vi "BALL-AND-BEAM.vi"() -> ()   [LabVIEW 2021]
uses:
  <vilib>/addons/control/pid/pid.llb/PID Structure.ctl
  <vilib>/addons/control/pid/pid.llb/PID Gain Unit.ctl
  <vilib>/addons/control/pid/pid.llb/PID Time Unit.ctl
  <vilib>/MakerHub/LINX/Public/Utilities/Open Serial.vi
  <vilib>/MakerHub/LINX/Public/Sensors/Motion/Servo/Servo Open One Channel.vi
  <vilib>/addons/control/pid/pid.llb/PID Structure Conversion (DBL).vi
  <vilib>/addons/control/pid/pid.llb/PID Advanced (DBL).vi
  <vilib>/MakerHub/LINX/Public/Sensors/Motion/Servo/Servo Set Pulse Width One Channel.vi
  <vilib>/MakerHub/LINX/Public/Sensors/Motion/Servo/Servo Close One Channel.vi
  <vilib>/MakerHub/LINX/LMH-LINX.lvlib
  <vilib>/MakerHub/LINX/Public/Sensors/Motion/Servo/Servo.lvlib
  <vilib>/MakerHub/LINX/Public/Sensors/Distance/Ultrasonic/Ultrasonic.lvlib
  <vilib>/ptbypt/NI_PtbyPt.lvlib
  <vilib>/addons/control/pid/NI_PID_pid.lvlib
panel:
  in  "auto? (T)":bool=TRUE
  out "XY Graph":cluster{"X":dbl, "Y":dbl}[](graph)
  in  "reinitialize? (F)":bool
  in  "manual control":dbl format="%.2f"
  out "BALL STABLE?":bool
  in  "output range":cluster{"output high":dbl, "output low":dbl}={"output high"=100.0, "output low"=-100.0} {"output low" format="%.2f"; "output high" format="%.2f"}
  out "Waveform Chart":cluster{"Dist":dbl, "Set Point":dbl}(graph)
  in  "setpoint range":cluster{"setpoint high":dbl, "setpoint low":dbl}={"setpoint high"=100.0, "setpoint low"=0.0} {"setpoint high" format="%.2f"; "setpoint low" format="%.2f"}
  out "PID OUTPUT":dbl
  in  "derivative unit":T1 items=["min", "s"]
  in  "integral unit":T1 items=["min", "s"]
  in  "derivative":dbl
  in  "integral":dbl
  in  "proportional":dbl
  in  "proportional unit":T2 items=["Gain (K)", "Band (PB)"]
  in  "PID structure":T3 items=["Academic (Standard)", "Parallel", "Series"]
  out "?":dbl(slide) scale=0.0..45.0
  out "?":dbl format="%0.2f"
  in  "TRIGGER_PIN":i32
  out "Loop Rate (Hz)":u32
  in  "Stop Bottom":bool
  out "?":dbl(slide) scale=0.0..45.0
  in  "ECHO_PIN":i32
  in  "?":dbl
  in  "Serial Port":refnum<visa-resource-name>="N/A"
  in  "Servo Pin":u32
  # "BALL AND BEAM"
  # "LINX Device Settings"
  # "Setpoint"
  # "Graph\nPID Gain"
  # "PID Configuration"
  # "Distance"
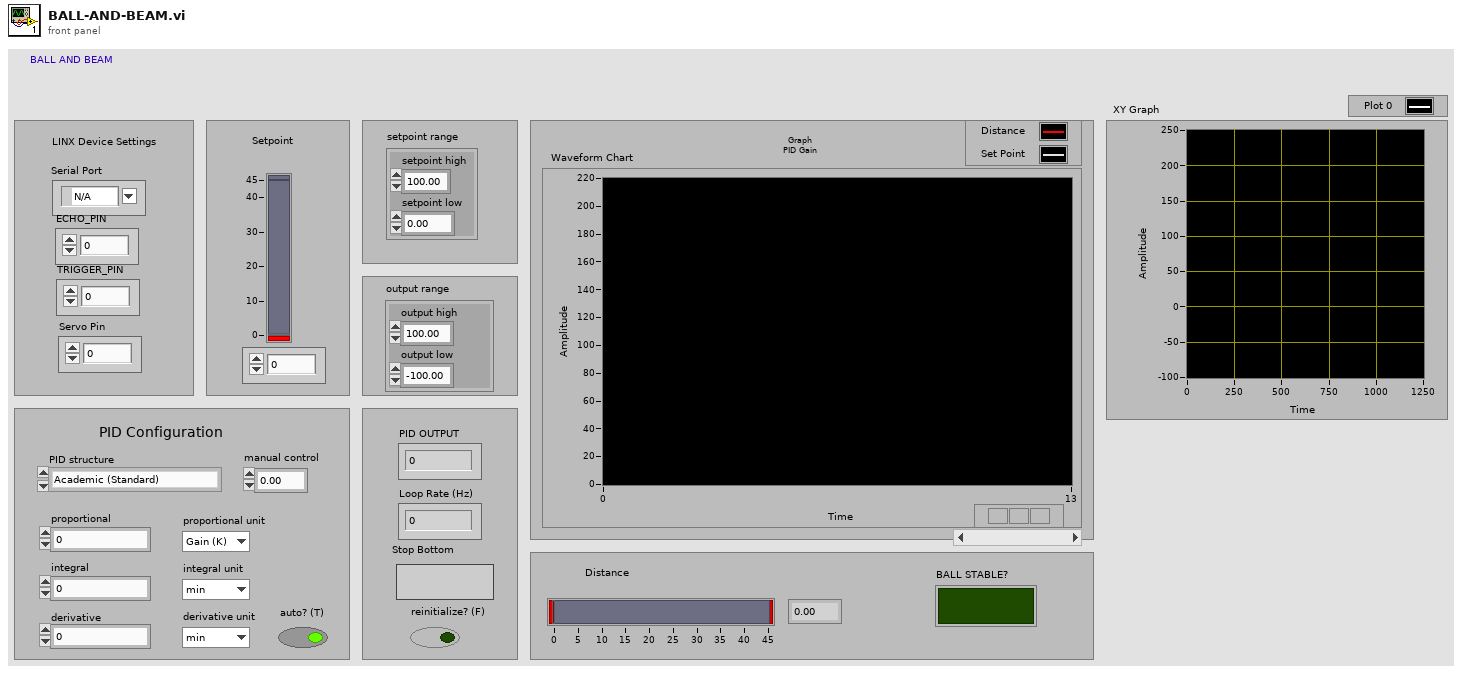
[diagram p1: front panel]
types:
  T1 = typedef "NI_PID_pid.lvlib/PID Time Unit.ctl" = u16
  T2 = typedef "NI_PID_pid.lvlib/PID Gain Unit.ctl" = u16
  T3 = typedef "NI_PID_pid.lvlib/PID Structure.ctl" = u16
  T4 = typedef "LMH-LINX.lvlib/LINX Ref.ctl" = cluster{"IO":T5, "Interface":T6, "LINX Device Config":T7}
  T5 = typedef "LMH-LINX.lvlib/Platform.ctl" = enum16{"Remote", "Local"}
  T6 = typedef "LMH-LINX.lvlib/Interface.ctl" = enum16{"Serial", "TCP"}
  T7 = typedef "LMH-LINX.lvlib/Device.lvlib/LINX Device Config.ctl" = cluster{"Interface":T6, "COM Port":refnum<visa-resource-name>, "TCP Configuration":T8, "Device Family":u8, "Device ID":u8, "Device Name":string, "TCP Ref":refnum<k5>, "Channels":T9}
  T8 = typedef "LMH-LINX.lvlib/Device.lvlib/TCP Config.ctl" = cluster{"IP Address":string, "Port":u16}
  T9 = typedef "LMH-LINX.lvlib/Channels.ctl" = cluster{"DI":u8[], "DO":u8[], "AI":u8[], "AO":u8[], "PWM":u8[], "QE":u8[], "UART":u8[], "I2C 2":u8[], "SPI":u8[], "CAN":u8[], "Servo":u8[], "AI Ref (V)":dbl, "AI Resolution (Bits)":u8, "AO Ref (V)":dbl, "AO Resolution (Bits)":u8}
  T10 = cluster{"proportional gain (Kc)":dbl, "integral time (Ti, min)":dbl, "derivative time (Td, min)":dbl}
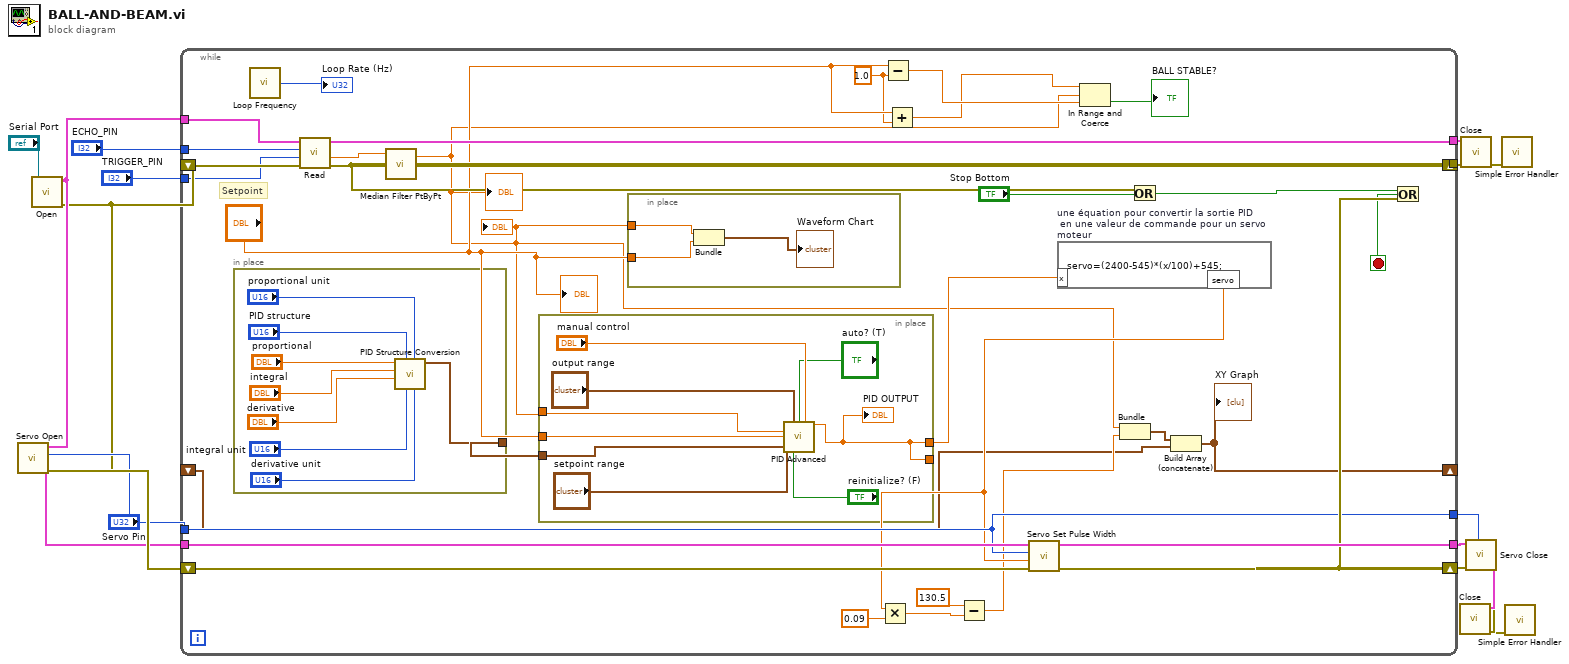
[diagram p0: block diagram]
diagram:
  n1 = call-poly <vilib>:"Open.vi"("Serial Port"="Serial Port") -> ("Error Out"=w3:errorcluster, "LINX Resource"=w14:T4)  [unwired: 8 in, 1 out]
  n2 = call-poly <vilib>:"Servo Open.vi"("Error In"=w3, "Servo Channel"="Servo Pin", "LINX Resource"=w14) -> ("Error Out"=w15:errorcluster, "LINX Resource"=w13:T4)  [unwired: 7 in]
  n3 = while {
    shift-right: [w40] -> _
    shift-left: w3 -> [w46]
    tunnel: w14 -> [w45]
    tunnel: "ECHO_PIN" -> [w44]
    shift-right: [w39] -> w8
    shift-left: w15 -> [w35]
    tunnel: w13 -> [w48]
    tunnel: "TRIGGER_PIN" -> [w43]
    tunnel: [w41] -> w11
    tunnel: [w40] -> w7
    tunnel: "Servo Pin" -> [w36]
    tunnel: [w36] -> w4
    tunnel: [w34] -> w2
    shift-right: [w19] -> _
    shift-left: _ -> [w18]
    stop <- w38 stop-if-true
    w30 = 1.0 ("y")
    # "Setpoint"
    n4 = in-place {
      in-place-border: [w59] -> w33
      n5 = call-poly <vilib>:"PID Structure Conversion.vi"("derivative unit"="derivative unit", "proportional unit"="proportional unit", "integral unit"="integral unit", "PID structure"="PID structure", "derivative"="derivative", "integral"="integral", "proportional"="proportional") -> ("PID gains"=w59:T10)  [unwired: 4 in]
    }
    n6 = call <vilib>:"Loop Frequency.vi"() -> ("Loop Rate (Hz)"=→"Loop Rate (Hz)":u32)
    n7 = call <vilib>:"Read.vi"("Error In"=w46, "DO Channel"=w43, "DI Channel"=w44, "LINX Resource"=w45) -> ("Error Out"=w40:errorcluster, "Centimeters"=w42:dbl, "LINX Resource"=w34:T4)  [unwired: 4 in, 1 out]
    n8 = call <vilib>:"Median Filter PtByPt.vi"("x"=w42) -> ("Filtered x"=w21:dbl)  [unwired: 3 in, 1 out]
    "?" <- w21
    "?" <- w21
    n9 = in-place {
      in-place-border: w33 -> [w58]
      in-place-border: [w51] -> w27
      in-place-border: "?" -> [w57]
      in-place-border: w21 -> [w56]
      in-place-border: [w51] -> _
      n10 = call-poly <vilib>:"PID Advanced.vi"("setpoint"=w57, "output range"="output range", "auto? (T)"="auto? (T)", "manual control"="manual control", "process variable"=w56, "setpoint range"="setpoint range", "PID gains"=w58, "reinitialize? (F)"="reinitialize? (F)") -> ("output"=w51:dbl)  [unwired: 6 in, 1 out]
      "PID OUTPUT" <- w51
    }
    n11 = in-place {
      in-place-border: "?" -> [w67]
      in-place-border: w21 -> [w68]
      n12 = Bundle("Filtered x"=w68, w67) -> (→"Waveform Chart":cluster{"Filtered x":dbl, dbl})  [unwired: 1 in]
    }
    n13 = Subtract(x="?", y=w30) -> (x-y=w29:dbl)
    n14 = Add(x="?", y=w30) -> (x+y=w28:dbl)
    n15 = formula code="servo=(2400-545)*(x/100)+545;" "une équation pour convertir la sortie PID\n en une valeur de commande pour un servo moteur"("x"=w27) -> ("servo"=w26:dbl)
    n16 = Multiply(x=w26, y=0.09) -> (x*y=w24:dbl)
    n17 = Subtract(x=130.5, y=w24) -> (x-y=w22:dbl)
    n18 = call-poly <vilib>:"Servo Set Pulse Width.vi"("Error In"=w35, "Pulse Width (uS)"=w26, "Servo Channel"=w36, "LINX Resource"=w48) -> ("Error Out"=w39:errorcluster, "LINX Resource"=w41:T4)  [unwired: 6 in]
    n19 = In Range and Coerce(upper limit=w28, x=w21, lower limit=w29) -> (In Range?=→"BALL STABLE?":bool)  [unwired: 1 out]
    n20 = Bundle("Filtered x"=w21, w22) -> (w20:cluster{"Filtered x":dbl, dbl})  [unwired: 1 in]
    n21 = Or(x=w40, y="Stop Bottom") -> (x .or. y?=w37:bool)
    n22 = Build Array (concatenate)(w20, w18) -> (w19:cluster{"Filtered x":dbl, dbl}[])
    "XY Graph" <- w19
    n23 = Or(x=w37, y=w39) -> (x .or. y?=w38:bool)
    "?" <- "?"
  }
  n24 = call <vilib>:"Close.vi"("Error In"=w7, "LINX Resource"=w2) -> ("Error Out"=w6:errorcluster)  [unwired: 9 in]
  n25 = call-poly <vilib>:"Servo Close.vi"("Error In"=w8, "Servo Channel"=w4, "LINX Resource"=w11) -> ("Error Out"=w9:errorcluster, "LINX Resource"=w10:T4)  [unwired: 7 in]
  n26 = call <vilib>:"Close.vi"("Error In"=w9, "LINX Resource"=w10) -> ("Error Out"=w1:errorcluster)  [unwired: 9 in]
  n27 = call <vilib>:"Simple Error Handler.vi"("error in (no error)"=w6) -> ()  [unwired: 4 in, 5 out]
  n28 = call <vilib>:"Simple Error Handler.vi"("error in (no error)"=w1) -> ()  [unwired: 4 in, 5 out]
